vi "Get Path.vi"(8 "error in (no error)":errorcluster, 11 "SequenceFile in":refnum<class "SequenceFile.lvclass">) -> (0 "error out":errorcluster, 2 "Path":path, 3 "SequenceFile out":refnum<class "SequenceFile.lvclass">)   [LabVIEW 2020, in "TSS.lvlib" / "SequenceFile.lvclass"]
uses:
  SequenceFile.lvclass
  SequenceFile.lvclass/SequenceFile.ctl
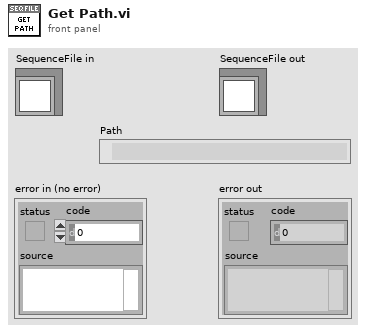
[diagram p1: front panel]
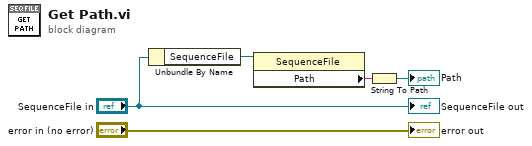
[diagram p0: block diagram]
diagram:
  n1 = Unbundle By Name("SequenceFile in") -> ("SequenceFile"=w3:refnum<k7>)
  n2 = property class="SequenceFile"(reference=w3) -> ("Path"=w2:string)  [unwired: 1 in, 2 out]
  n3 = String To Path(string=w2) -> (path=→"Path":path)
  "error out" <- "error in (no error)"
  "SequenceFile out" <- "SequenceFile in"
